vi "PF200_6_24.vi"() -> ()   [LabVIEW 2020]
uses:
  <vilib>/DAQmx/read.llb/DAQmx Read (Analog 1D DBL NChan 1Samp).vi
  <vilib>/DAQmx/read.llb/DAQmx Read (Analog DBL 1Chan 1Samp).vi
  <vilib>/DAQmx/create/channels.llb/DAQmx Create Channel (AI-Voltage-Basic).vi
  <vilib>/DAQmx/miscellaneous.llb/DAQmx Fill In Error Info.vi
  <vilib>/Utility/file.llb/Write Delimited Spreadsheet (string).vi
  <vilib>/Utility/file.llb/Write Delimited Spreadsheet (DBL).vi
panel:
  out "Waveform Chart":dbl(graph)
  in  "dev1 physical channels 2":tag
  out "Elapsed time (sec)":dbl
  out "XY Graph":cluster{dbl[], dbl[]}[](graph)
  in  "Seconds per data point (sec)":dbl
  in  "stop":bool
  in  "dev1 physical channels":tag
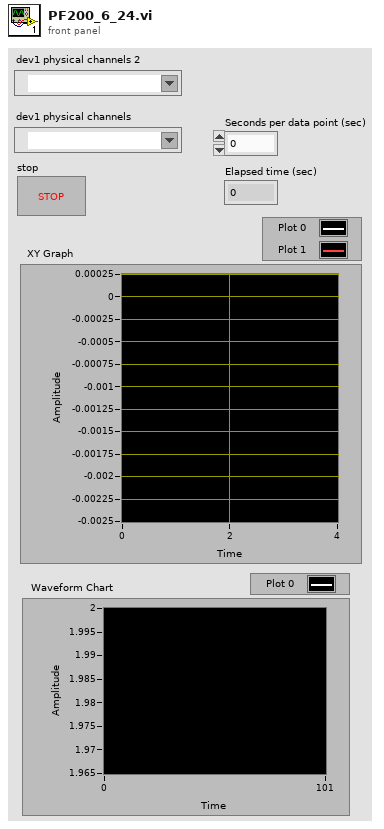
[diagram p1: front panel]
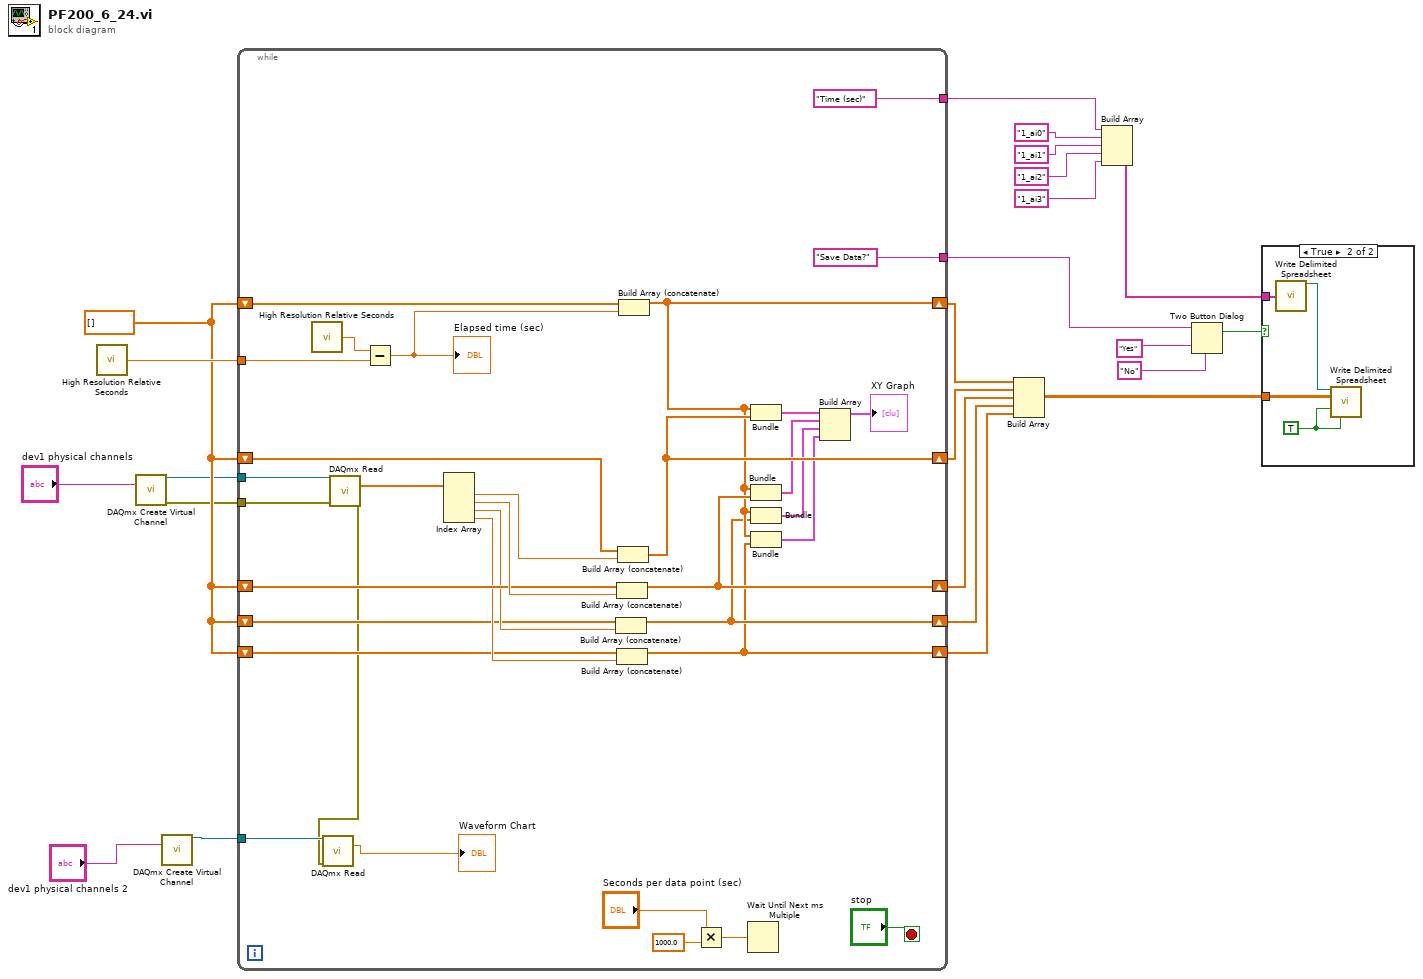
[diagram p0: block diagram]
diagram:
  w21 = dbl[] []
  n1 = call <vilib>:"High Resolution Relative Seconds.vi"() -> ("relative seconds"=w22:dbl)
  n2 = call-poly <vilib>:"DAQmx Create Virtual Channel.vi"("physical channels"="dev1 physical channels") -> ("task out"=w20:refnum<k21>, "error out"=w19:errorcluster)  [unwired: 13 in]
  n3 = call-poly <vilib>:"DAQmx Create Virtual Channel.vi"("physical channels"="dev1 physical channels 2") -> ("task out"=w11:refnum<k21>)  [unwired: 13 in, 1 out]
  n4 = while {
    tunnel: w22 -> [w53]
    shift-right: [w36] -> w18
    shift-left: w21 -> [w50]
    shift-right: [w44] -> w17
    shift-left: w21 -> [w47]
    shift-right: [w43] -> w16
    shift-left: w21 -> [w45]
    shift-right: [w34] -> w15
    shift-left: w21 -> [w38]
    shift-right: [w33] -> w14
    shift-left: w21 -> [w37]
    tunnel: w20 -> [w30]
    tunnel: w19 -> [w29]
    tunnel: w11 -> [w28]
    tunnel: ["Time (sec)"] -> w5
    tunnel: ["Save Data?" ("message")] -> w1
    stop <- "stop" stop-if-true
    n5 = call <vilib>:"High Resolution Relative Seconds.vi"() -> ("relative seconds"=w52:dbl)
    n6 = call-poly <vilib>:"DAQmx Read.vi"("task/channels in"=w30, "error in"=w29) -> ("data"=w49:dbl[], "error out"=w26:errorcluster)  [unwired: 11 in, 1 out]
    n7 = call-poly <vilib>:"DAQmx Read.vi"("task/channels in"=w28, "error in"=w26) -> ("data"=→"Waveform Chart":dbl)  [unwired: 11 in, 2 out]
    n8 = Subtract(x=w52, y=w53) -> (x-y=w51:dbl)
    "Elapsed time (sec)" <- w51
    n9 = Index Array(array=w49) -> (element #1=w48:dbl, element #2=w46:dbl, element #3=w40:dbl, element #4=w39:dbl)  [unwired: 4 in]
    n10 = Build Array (concatenate)(w38, w40) -> (w34:dbl[])
    n11 = Build Array (concatenate)(w45, w46) -> (w43:dbl[])
    n12 = Build Array (concatenate)(w37, w39) -> (w33:dbl[])
    n13 = Build Array (concatenate)(w47, w48) -> (w44:dbl[])
    n14 = Build Array (concatenate)(w50, w51) -> (w36:dbl[])
    n15 = Multiply(x="Seconds per data point (sec)", y=1000.0) -> (x*y=w56:dbl)
    n16 = Wait Until Next ms Multiple(millisecond multiple=w56) -> ()  [unwired: 1 out]
    n17 = Bundle(w36, w44) -> (w35:cluster{dbl[], dbl[]})  [unwired: 1 in]
    n18 = Bundle(w36, w43) -> (w42:cluster{dbl[], dbl[]})  [unwired: 1 in]
    n19 = Bundle(w36, w34) -> (w32:cluster{dbl[], dbl[]})  [unwired: 1 in]
    n20 = Bundle(w36, w33) -> (w31:cluster{dbl[], dbl[]})  [unwired: 1 in]
    n21 = Build Array(w35, w42, w32, w31) -> (→"XY Graph":cluster{dbl[], dbl[]}[])
  }
  n22 = Build Array(w18, w17, w16, w15, w14) -> (w13:dbl[][])
  n23 = Build Array(w5, "1_ai0", "1_ai1", "1_ai2", "1_ai3") -> (w6:string[])
  n24 = Two Button Dialog(message=w1, 1:"No" ("F button name (\"Cancel\")"), 2:"Yes" ("T button name (\"OK\")")) -> (T button?=w4:bool)
  n25 = case shown="True" w4 {
    tunnel: w13 -> [_ w61]
    tunnel: w6 -> [_ w60]
    frame False {
    }
    frame True {
      w58 = TRUE ("transpose? (no:F)")
      n26 = call-poly <vilib>:"Write Delimited Spreadsheet.vi"("1D data"=w60) -> ("new file path (Not A Path if cancelled)"=w59:path)  [unwired: 13 in, 1 out]
      n27 = call-poly <vilib>:"Write Delimited Spreadsheet.vi"("file path (dialog if empty)"=w59, "2D data"=w61, "append to file? (new file:F)"=w58, "transpose? (no:F)"=w58) -> ()  [unwired: 10 in, 2 out]
    }
  }
